vi "test-TimeInterpRotation-Test1.vi"() -> (3 "All tests passed":bool)   [LabVIEW 2019]
uses:
  <vilib>/Rock Robotics/WPI/ThirdParty/JAS_Junk/TrajLib/ROTATION2D.ctl
  <vilib>/Rock Robotics/WPI/ThirdParty/JAS_Junk/TrajLib/Util_CalcDist.vi
  <vilib>/Rock Robotics/WPI/ThirdParty/JAS_Junk/TrajLib/TimeInterpRotation_CleanUp.vi
  <vilib>/gmath/interp.llb/Search Ordered Table.vi
  <vilib>/Rock Robotics/WPI/ThirdParty/JAS_Junk/TrajLib/Trajectory_Library.lvlib
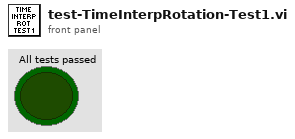
[diagram p1: front panel]
types:
  T1 = typedef "Trajectory_Library.lvlib/ROTATION2D.ctl" = cluster{"VALUE":dbl, "COS":dbl, "SIN":dbl}
  T2 = typedef "Trajectory_Library.lvlib/TIME_INTERPOLATABLE_ROTATION.ctl" = cluster{"TimeStamps":dbl[], "RotationValues":T1[], "Min_TimeStamp":dbl, "Max_TimeStamp":dbl, "ItemCount":i32, "MaxBufferTime":dbl}
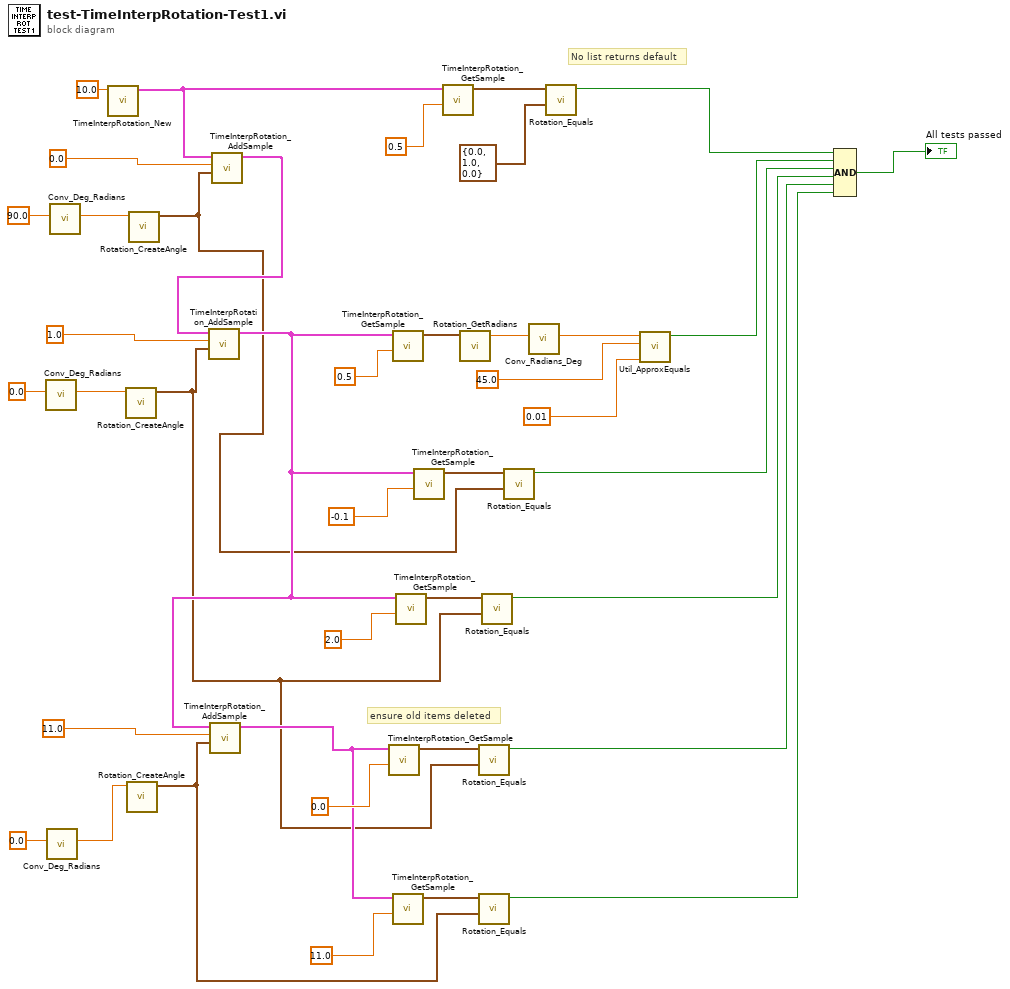
[diagram p0: block diagram]
diagram:
  # "ensure old items deleted"
  # "No list returns default"
  n1 = call <vilib>:"Conv_Deg_Radians.vi"("Degress"=0.0) -> ("Radians"=w6:dbl)  [unwired: 10 in]
  n2 = call <vilib>:"Conv_Deg_Radians.vi"("Degress"=0.0) -> ("Radians"=w7:dbl)  [unwired: 10 in]
  n3 = call <vilib>:"Conv_Deg_Radians.vi"("Degress"=90.0) -> ("Radians"=w5:dbl)  [unwired: 10 in]
  n4 = call <vilib>:"TimeInterpRotation_New.vi"("MaxTime"=10.0) -> ("TimeInterpRotation"=w27:T2)  [unwired: 10 in]
  n5 = call <vilib>:"Rotation_CreateAngle.vi"("Angle"=w6) -> ("ROTATION"=w8:T1)  [unwired: 10 in]
  n6 = call <vilib>:"Rotation_CreateAngle.vi"("Angle"=w7) -> ("ROTATION"=w11:T1)  [unwired: 10 in]
  n7 = call <vilib>:"Rotation_CreateAngle.vi"("Angle"=w5) -> ("ROTATION"=w4:T1)  [unwired: 10 in]
  n8 = call <vilib>:"TimeInterpRotation_AddSample.vi"("RotationValue"=w4, "TimeStamp"=0.0, "in TimeInterpRotation"=w27) -> ("out TimeInterpRotation"=w29:T2)  [unwired: 7 in, 1 out]
  n9 = call <vilib>:"TimeInterpRotation_AddSample.vi"("RotationValue"=w8, "TimeStamp"=1.0, "in TimeInterpRotation"=w29) -> ("out TimeInterpRotation"=w17:T2)  [unwired: 7 in, 1 out]
  n10 = call <vilib>:"TimeInterpRotation_AddSample.vi"("RotationValue"=w11, "TimeStamp"=11.0, "in TimeInterpRotation"=w17) -> ("out TimeInterpRotation"=w12:T2)  [unwired: 7 in, 1 out]
  n11 = call <vilib>:"TimeInterpRotation_GetSample.vi"("TimeStamp"=0.0, "TimeInterpRotation"=w12) -> ("OutputRotation"=w15:T1)  [unwired: 9 in]
  n12 = call <vilib>:"TimeInterpRotation_GetSample.vi"("TimeStamp"=0.5, "TimeInterpRotation"=w17) -> ("OutputRotation"=w3:T1)  [unwired: 9 in]
  n13 = call <vilib>:"TimeInterpRotation_GetSample.vi"("TimeStamp"=11.0, "TimeInterpRotation"=w12) -> ("OutputRotation"=w13:T1)  [unwired: 9 in]
  n14 = call <vilib>:"TimeInterpRotation_GetSample.vi"("TimeStamp"=2.0, "TimeInterpRotation"=w17) -> ("OutputRotation"=w22:T1)  [unwired: 9 in]
  n15 = call <vilib>:"TimeInterpRotation_GetSample.vi"("TimeStamp"=-0.1, "TimeInterpRotation"=w17) -> ("OutputRotation"=w24:T1)  [unwired: 9 in]
  n16 = call <vilib>:"TimeInterpRotation_GetSample.vi"("TimeStamp"=0.5, "TimeInterpRotation"=w27) -> ("OutputRotation"=w28:T1)  [unwired: 9 in]
  n17 = call <vilib>:"Rotation_GetRadians.vi"("in ROTATION"=w3) -> ("AngleRadians"=w2:dbl)  [unwired: 10 in]
  n18 = call <vilib>:"Rotation_Equals.vi"("other ROTATION"=w8, "in ROTATION"=w15) -> ("Equals"=w10:bool)  [unwired: 9 in]
  n19 = call <vilib>:"Rotation_Equals.vi"("other ROTATION"=w11, "in ROTATION"=w13) -> ("Equals"=w9:bool)  [unwired: 9 in]
  n20 = call <vilib>:"Rotation_Equals.vi"("other ROTATION"=w8, "in ROTATION"=w22) -> ("Equals"=w20:bool)  [unwired: 9 in]
  n21 = call <vilib>:"Rotation_Equals.vi"("other ROTATION"=w4, "in ROTATION"=w24) -> ("Equals"=w21:bool)  [unwired: 9 in]
  n22 = call <vilib>:"Conv_Radians_Deg.vi"("Radians"=w2) -> ("Degrees"=w34:dbl)  [unwired: 10 in]
  n23 = call <vilib>:"Rotation_Equals.vi"("other ROTATION"=T1 {"VALUE"=0.0, "COS"=1.0, "SIN"=0.0} ("ROTATION"), "in ROTATION"=w28) -> ("Equals"=w1:bool)  [unwired: 9 in]
  n24 = call <vilib>:"Util_ApproxEquals.vi"("Tolerance"=0.01, "Value 2"=45.0, "Value 1"=w34) -> ("ApproxEquals"=w31:bool)  [unwired: 8 in]
  n25 = Compound Arithmetic op=AND(w1, w31, w21, w20, w10, w9) -> (→"All tests passed":bool)
